vi "Real Lorentzian Function.vi"(3 "output control":T1, 4 "data":variant, 5 "X":dbl[](array[numeric]), 6 "a":dbl[](array[numeric])) -> (0 "error out":errorcluster, 1 "f'(X,a)":dbl[][](array[numeric]), 2 "f(X,a)":dbl[](array[numeric]))   [LabVIEW 2016]
doc: "Sum of three Gaussians, plus DC offset."
uses:
  <vilib>/gmath/NumericalOptimization/LM_output select.ctl
  <vilib>/gmath/NI_Gmath.lvlib
panel:
  out "Waveform Graph":dbl[](graph)
  # "F0\nG\nA"
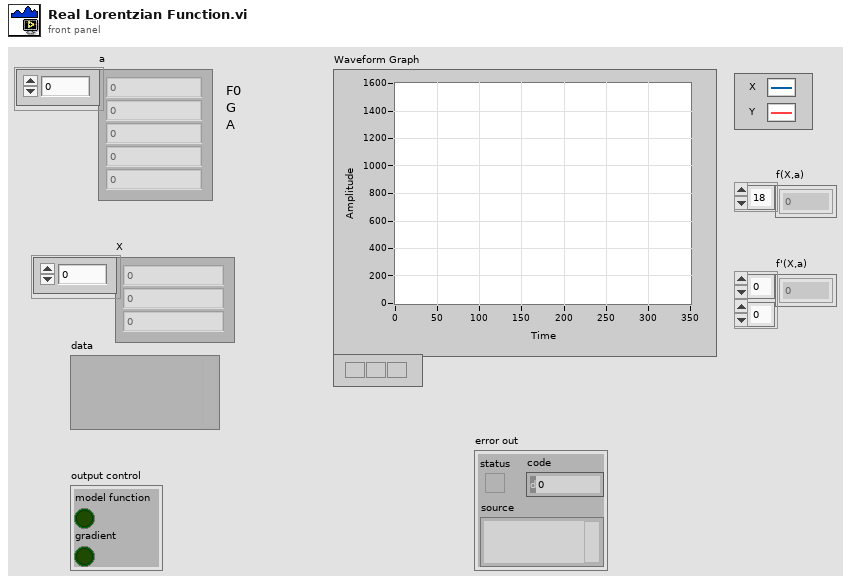
[diagram p1: front panel]
types:
  T1 = typedef "NI_Gmath.lvlib/LM_output select.ctl" = cluster{"model function":bool, "gradient":bool}
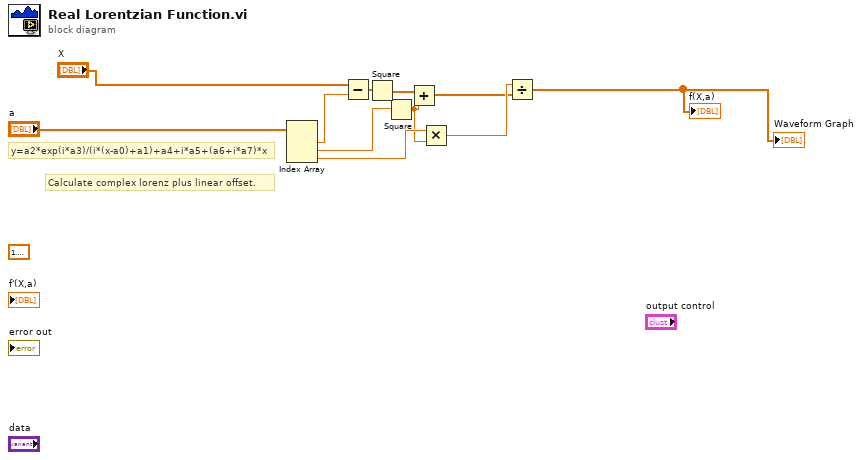
[diagram p0: block diagram]
diagram:
  (unwired) 1.5707963267948966
  # "y=a2*exp(i*a3)/(i*(x-a0)+a1)+a4+i*a5+(a6+i*a7)*x"
  # "Calculate complex lorenz plus linear offset."
  n1 = Index Array(array="a") -> (element #1=w10:dbl, element #2=w7:dbl, element #3=w5:dbl)  [unwired: 3 in]
  n2 = Subtract(x="X", y=w10) -> (x-y=w8:dbl[])
  n3 = Square(x=w8) -> (x^2=w6:dbl[])
  n4 = Square(x=w7) -> (x^2=w1:dbl)
  n5 = Add(x=w6, y=w1) -> (x+y=w3:dbl[])
  n6 = Multiply(x=w5, y=w1) -> (x*y=w4:dbl)
  n7 = Divide(x=w4, y=w3) -> (x/y=→"f(X,a)" →"Waveform Graph":dbl[])
